vi "LVClass_WavefrontCorrectorSet ctor.vi"(0 "WavefrontCorrectorSet (const)":refnum<class "WavefrontCorrectorSet.lvclass">, 5 "PathToWavefrontCorrectorSetupFile":path, 11 "error in (no error)":errorcluster) -> (4 "WavefrontCorrectorSet (new)":refnum<class "WavefrontCorrectorSet.lvclass">, 15 "error out":errorcluster)   [LabVIEW 2020, in "WavefrontCorrectorSet.lvclass"]
doc: "WavefrontCorrectorSet constructor.\n\n--------------------------------------------------------------------------------\n\n<B>wavefrontcorrector_setIn </B> : Constant Pointer to WavefrontCorrectorSet object.\n<B>wavefrontcorrector_setOut </B> : Constant Pointer to WavefrontCorrectorSet object.\n<B>config_file_path </B> : Absolute path to Haso or Camera configuration file.\n<B>ErrorIn </B> : Error\n<B>ErrorOut </B> : Error\n\n--------------------------------------------------------------------------------"
uses:
  WavefrontCorrectorSet.lvclass
  Handle creation.ctl
  WavefrontCorrectorSet.lvclass/WavefrontCorrectorSet.ctl
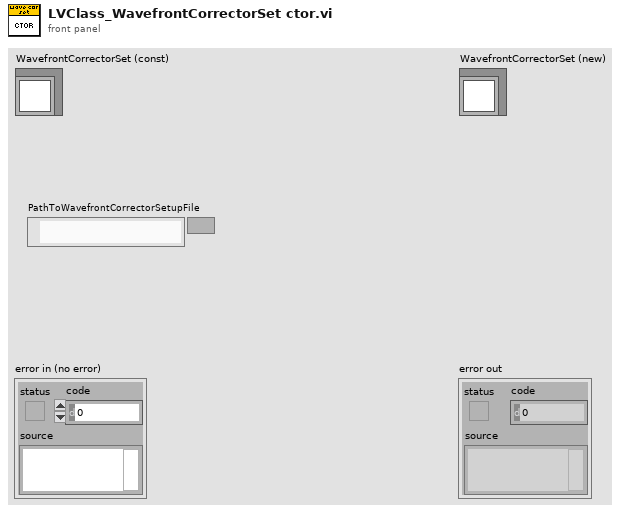
[diagram p1: front panel]
types:
  T1 = typedef "Handle creation.ctl" = enum16{"By ctor", "By write function"}
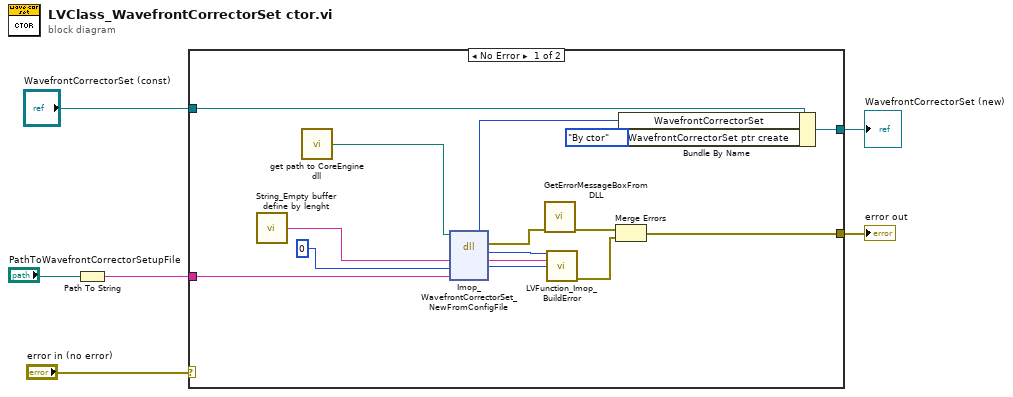
[diagram p0: block diagram]
diagram:
  n1 = Path To String(path="PathToWavefrontCorrectorSetupFile") -> (string=w2:string)
  n2 = case shown="No Error" "error in (no error)" {
    selector: "error in (no error)" -> [_ w22]
    tunnel: [w10 w22] -> w3
    tunnel: [w13 w21] -> w4
    tunnel: "WavefrontCorrectorSet (const)" -> [w14 w21]
    tunnel: w2 -> [w9 _]
    frame No Error {
      n3 = call "String_Empty buffer define by lenght.vi"() -> ("Empty buffer"=w20:string)  [unwired: 1 in]
      n4 = call "get path to CoreEngine dll.vi"() -> ("path to wavekit library"=w8:path)  [unwired: 14 in, 1 out]
      n5 = dll-call lib="D:/soft/HASO_v3/SVN_trunk/ImOpCoreEngine4_LV2011/DLLs/c_interface_vc100.dll" fn="Imop_WavefrontCorrectorSet_NewFromConfigFile"(path in=w8, "message"=w20, "WavefrontCorrectorSet"=0 ("Pupil"), "Config_file_path"=w9) -> (error out=w17:errorcluster, "return type"=w18:i32, "message"=w19:string, "WavefrontCorrectorSet"=w7:i64)  [unwired: 3 in, 1 out]
      n6 = call "GetErrorMessageBoxFromDLL.vi"("error IN"=w17) -> ("error OUT"=w12:errorcluster)  [unwired: 10 in]
      n7 = call "LVFunction_Imop_BuildError.vi"("code"=w18, "String to Prepend to source (\"\")"=w19, "Adresse"=w7) -> ("error out"=w11:errorcluster)  [unwired: 12 in]
      n8 = Merge Errors(w12, w11) -> (w10:errorcluster)
      n9 = Bundle By Name(cluster=w14, "WavefrontCorrectorSet"=w7, "WavefrontCorrectorSet ptr create"=Handle_creation."By ctor" ("Pupil ptr create")) -> (w13:refnum<class "WavefrontCorrectorSet.lvclass">)
    }
    frame Error {
    }
  }
  "error out" <- w3
  "WavefrontCorrectorSet (new)" <- w4
